vi "InsertItem.vi"(7 "Parent Tag":string, 8 "error in (no error)":errorcluster, 10 "MenuItem":refnum<class "MGI_MenuItem.lvclass">, 11 "MGI_Control in":refnum<class "MGI_Control.lvclass">) -> (0 "error out":errorcluster, 3 "MGI_Control out":refnum<class "MGI_Control.lvclass">)   [LabVIEW 2016, in "MGI_Control.lvclass"]
doc: "Authored by Derek E. Trepanier\nsupport@mooregoodideas.com\nwww.mooregoodideas.com\n\nCopyright (c) 2012, Moore Good Ideas, Inc.\n\nAll rights reserved.\n\nRedistribution and use in source and binary forms, with or without modification, are permitted provided that the following conditions are met:\n\n * Redistributions of source code must retain the above copyright notice, this list of conditions and the following disclaimer.\n * Redistributions in binary form must reproduce the above copyright notice, this list of conditions and the following disclaimer in the documentation and/or other materials provided with the distribution.\n * Neither the name of Moore Good Ideas, Inc. nor the names of its contributors may be used to endorse or promote products derived from this software without specific prior written permission.\n\nTHIS SOFTWARE IS PROVIDED BY THE COPYRIGHT HOLDERS AND CONTRIBUTORS \"AS IS\" AND ANY EXPRESS OR IMPLIED WARRANTIES, INCLUDING, BUT NOT LIMITED TO, THE IMPLIED WARRANTIES OF MERCHANTABILITY AND FITNESS FOR A PARTICULAR PURPOSE ARE DISCLAIMED. IN NO EVENT SHALL THE COPYRIGHT OWNER OR CONTRIBUTORS BE LIABLE FOR ANY DIRECT, INDIRECT, INCIDENTAL, SPECIAL, EXEMPLARY, OR CONSEQUENTIAL DAMAGES (INCLUDING, BUT NOT LIMITED TO, PROCUREMENT OF SUBSTITUTE GOODS OR SERVICES; LOSS OF USE, DATA, OR PROFITS; OR BUSINESS INTERRUPTION) HOWEVER CAUSED AND ON ANY THEORY OF LIABILITY, WHETHER IN CONTRACT, STRICT LIABILITY, OR TORT (INCLUDING NEGLIGENCE OR OTHERWISE) ARISING IN ANY WAY OUT OF THE USE OF THIS SOFTWARE, EVEN IF ADVISED OF THE POSSIBILITY OF SUCH DAMAGE."
uses:
  <userlib>/_MGI/Menu Building/MenuTypes/Control/MGI_Control.lvclass
  <userlib>/_MGI/Menu Building/MenuItem/MGI_MenuItem.lvclass
  <userlib>/_MGI/Menu Building/MenuTypes/Control/MGI_Control.lvclass/MGI_Control.ctl
  <userlib>/_MGI/Menu Building/MenuItem/Read Full Tag.vi
  <userlib>/_MGI/Menu Building/MenuItem/Read Enabled.vi
  <userlib>/_MGI/Menu Building/MenuItem/Read Checked.vi
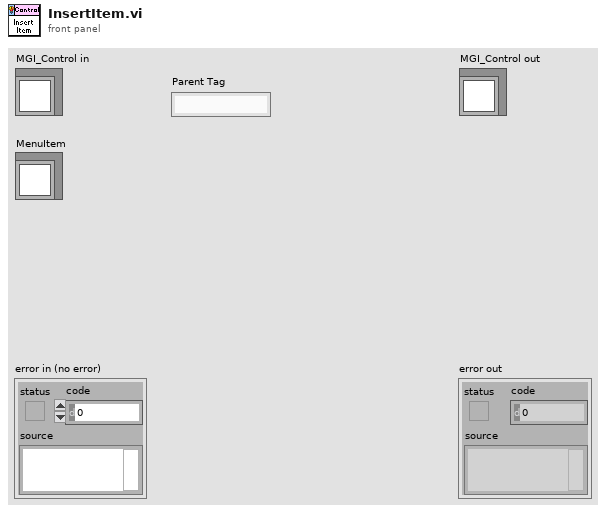
[diagram p1: front panel]
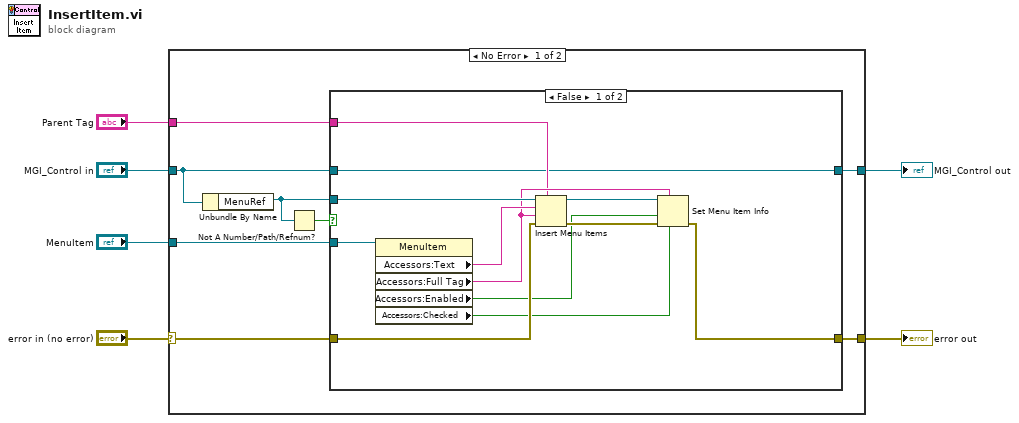
[diagram p0: block diagram]
diagram:
  n1 = case shown="No Error" "error in (no error)" {
    selector: "error in (no error)" -> [w12 w30]
    tunnel: [w11 w30] -> w1
    tunnel: [w10 w29] -> w2
    tunnel: "MGI_Control in" -> [w9 w29]
    tunnel: "Parent Tag" -> [w14 _]
    tunnel: "MenuItem" -> [w13 _]
    frame No Error {
      n2 = Unbundle By Name(w9) -> ("MenuRef"=w8:refnum<k9>)
      n3 = Not A Number/Path/Refnum?(number/path/refnum=w8) -> (NaN/Path/Refnum?=w7:bool)
      n4 = case shown="False" w7 {
        tunnel: w8 -> [w26 _]
        tunnel: w14 -> [w19 _]
        tunnel: w13 -> [w25 _]
        tunnel: w12 -> [w23 w27]
        tunnel: [w17 w27] -> w11
        tunnel: [w18 w28] -> w10
        tunnel: w9 -> [w18 w28]
        frame False {
          n5 = property class="MenuItem"(reference=w25) -> ("Accessors:Text"=w24:string, "Accessors:Full Tag"=w20:string, "Accessors:Enabled"=w16:bool, "Accessors:Checked"=w15:bool)  [unwired: 1 in, 2 out]
          n6 = Insert Menu Items(5:w19, 6:w23, 7:w20, 8:w24, 9:w26) -> (0:w21:errorcluster, 3:w22:refnum<k9>)  [unwired: 1 in, 1 out]
          n7 = Set Menu Item Info(6:w15, 7:w20, 8:w21, 9:w16, 11:w22) -> (0:w17:errorcluster)  [unwired: 2 in, 1 out]
        }
        frame True {
        }
      }
    }
    frame Error {
    }
  }
  "error out" <- w1
  "MGI_Control out" <- w2
